vi "wait.vi"(0 "HGF_NextMultiple":refnum<class "HGF_Wait.lvclass">, 3 "msTimeout (-1)":i32=-1, 5 "error in (no error)":errorcluster, 9 "ignore previous (F)":bool) -> (14 "dup HGF_NextMultiple":refnum<class "HGF_Wait.lvclass">, 16 "Object":refnum<class>, 17 "timed out":bool, 19 "error out":errorcluster)   [LabVIEW 2014, in "HGF_BaseClasses.lvlib" / "HGF_Wait.lvclass"]
doc: "Use this VI to wait for a time specified in timeout value."
uses:
  HGF_Wait.lvclass
  HGF_Event/HGF_Event.lvclass
  HGF_Timing/HGF_Timing.lvclass
  HGF_Auxiliary/Severity.ctl
  HGF_Auxiliary/HGF_Auxiliary.lvlib
  HGF_Auxiliary/ErrorCode.ctl
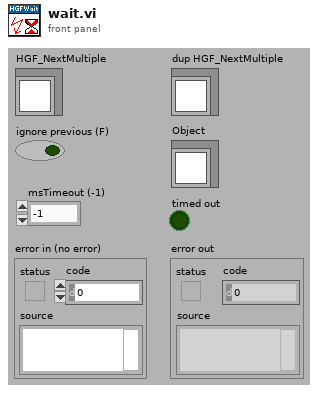
[diagram p1: front panel]
types:
  T1 = typedef "HGF_Auxiliary.lvlib/ErrorCode.ctl" = enum32{"No error", "Function not supported.", "This VI is for friends only.", "Reference object aready exisits.", "Parameter out of range.", "Not a rendezvous.", "Invalid notifier reference.", "Invalid queue reference.", "Self-Test not supported.", "Reset not supported.", "IDN query not supported.", "Error query not supported.", "Incorrect addressee.", "Object already exists.", "No class name specified", "Driver not supported", "Attribute is not writable"}
  T2 = typedef "HGF_Auxiliary.lvlib/Severity.ctl" = enum16{"Info", "Warning", "Fault", "Error", "Fatal"}
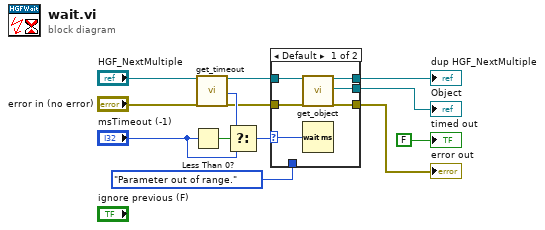
[diagram p0: block diagram]
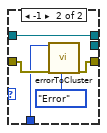
[diagram p2: hidden frame]
diagram:
  n1 = Less Than 0?(x="msTimeout (-1)") -> (x < 0?=w10:bool)
  n2 = call "get_timeout.vi"("HGF_Event.lvclass in"="HGF_NextMultiple", "error in (no error)"="error in (no error)") -> ("HGF_Event.lvclass out"=w7:refnum<class "HGF_Wait.lvclass">, "timeout"=w9:i32, "error out"=w6:errorcluster)  [unwired: 15 out]
  n3 = Select(t=w9, s=w10, f="msTimeout (-1)") -> (s? t:f=w1:i32)
  n4 = case shown="Default" w1 {
    selector: w1 -> [w14 _]
    tunnel: [w17 w24] -> w5
    tunnel: [w15 _] -> w4
    tunnel: [w16 w22] -> w3
    tunnel: w7 -> [w19 w24]
    tunnel: w6 -> [w18 w23]
    tunnel: ErrorCode."Parameter out of range." ("error code") -> [_ w20]
    frame Default {
      n5 = call "get_object.vi"("HGF_Timing.lvclass"=w19, "error in (no error)"=w18) -> ("dup HGF_Timing"=w17:refnum<class "HGF_Wait.lvclass">, "object"=w15:refnum<class>, "error out"=w16:errorcluster)  [unwired: 15 out]
      n6 = Wait (ms)(milliseconds to wait=w14) -> ()  [unwired: 1 out]
    }
    frame -1 {
      n7 = call "errorToCluster.vi"("error code"=w20, "error in (no error)"=w23, "severity (Error)"=Severity."Error") -> ("error out"=w22:errorcluster)  [unwired: 2 in, 14 out]
    }
  }
  "error out" <- w3
  "dup HGF_NextMultiple" <- w5
  "Object" <- w4
  "timed out" <- FALSE ("timed out")
